vi "add search path.vi"(6 "include llb (T)":bool=TRUE, 8 "error in":errorcluster, 9 "exclusions":string[](array[string]), 10 "Path":path, 11 "vi modification tool in":refnum<class "VI modification collection.lvclass">) -> (0 "error out":errorcluster, 3 "vi modification tool out":refnum<class "VI modification collection.lvclass">)   [LabVIEW 2013, in "VI modification collection.lvclass"]
uses:
  VI modification collection.lvclass
  VI modification collection.lvclass/VI modification collection.ctl
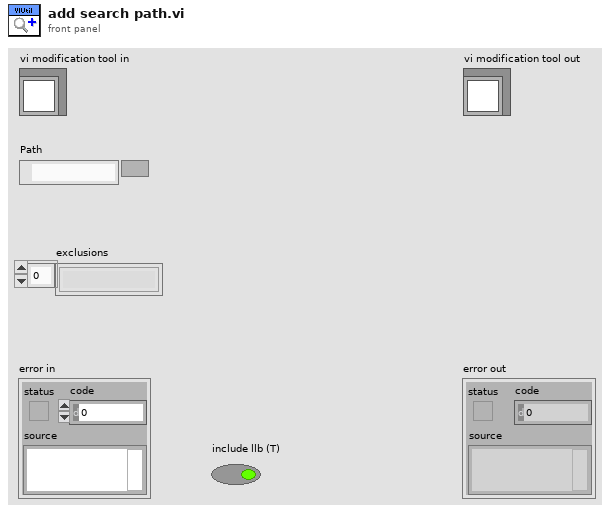
[diagram p1: front panel]
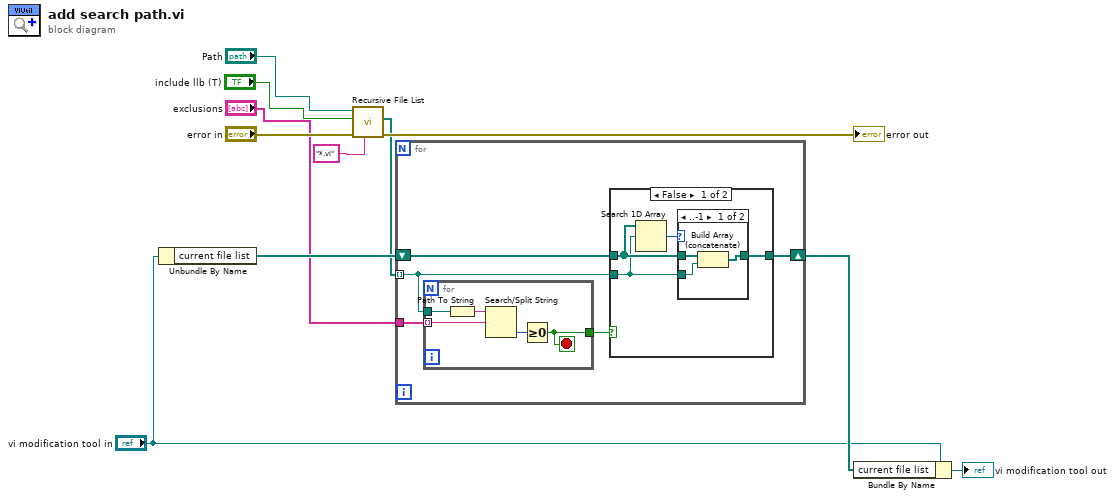
[diagram p0: block diagram]
diagram:
  n1 = Unbundle By Name("vi modification tool in") -> ("current file list"=w10:path[])
  n2 = call <vilib>:"Recursive File List.vi"("pattern"="*.vi", "error in (no error)"="error in", "Treat LLBs as Folders?"="include llb (T)", "Folder Path"="Path") -> ("error out"=→"error out":errorcluster, "All Files in Dir"=w2:path[])  [unwired: 3 in, 3 out]
  n3 = for {
    tunnel: w2 -> [w12] mode=indexing
    tunnel: "exclusions" -> [w16]
    shift-right: [w14] -> w11
    shift-left: w10 -> [w13]
    n4 = for {
      tunnel: w12 -> [w26]
      tunnel: w16 -> [w30] mode=indexing
      tunnel: [w28] -> w15
      stop <- w28 stop-if-true
      n5 = Path To String(path=w26) -> (string=w27:string)
      n6 = Search/Split String(string=w27, search string/char (-)=w30) -> (offset of match=w29:i32)  [unwired: 1 in, 2 out]
      n7 = Greater Or Equal To 0?(x=w29) -> (x >= 0?=w28:bool)
    }
    n8 = case shown="False" w15 {
      tunnel: [w19 w25] -> w14
      tunnel: w13 -> [w18 w25]
      tunnel: w12 -> [w17 _]
      frame False {
        n9 = Search 1D Array(1D array=w18, element=w17) -> (index of element=w20:i32)  [unwired: 1 in]
        n10 = case shown="..-1" w20 {
          tunnel: [w21 w24] -> w19
          tunnel: w18 -> [w22 w24]
          tunnel: w17 -> [w23 _]
          frame ..-1 {
            n11 = Build Array (concatenate)(w22, w23) -> (w21:path[])
          }
          frame 0.. {
          }
        }
      }
      frame True {
      }
    }
  }
  n12 = Bundle By Name(cluster="vi modification tool in", "current file list"=w11) -> (→"vi modification tool out":refnum<class "VI modification collection.lvclass">)
